vi "ReadDictionary.vi"(8 "error in (no error)":errorcluster, 11 "Dictionary File Path":path) -> (0 "error out":errorcluster, 1 "CSV String":string, 2 "Dictionary":T1, 3 "Dictionary File Path out":path)   [LabVIEW 2020]
uses:
  Dictionary--Cluster.ctl
  Font -- Cluster.ctl
  Phrase Dictionary Entry -- Cluster.ctl
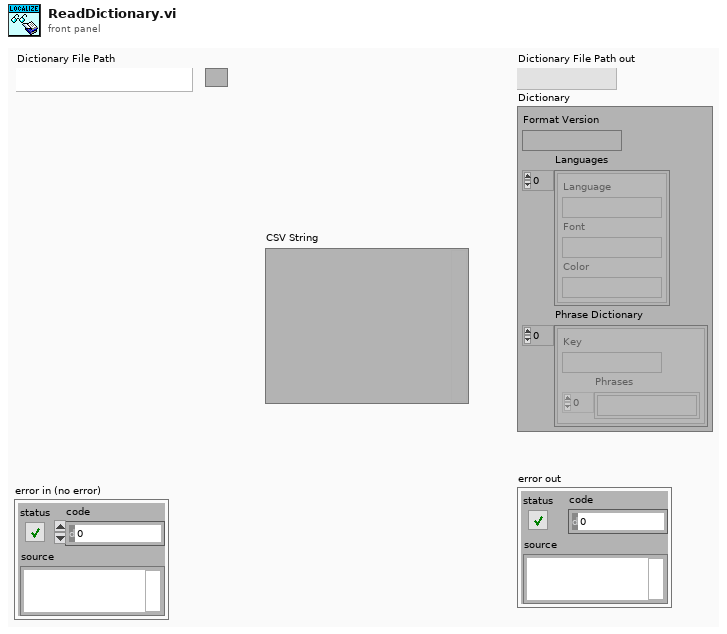
[diagram p1: front panel]
types:
  T1 = typedef "Dictionary--Cluster.ctl" = cluster{"Format Version":string, "Languages":T2[], "Phrase Dictionary":T3[]}
  T2 = typedef "Font -- Cluster.ctl" = cluster{"Language":string, "Font":string, "Color":string}
  T3 = typedef "Phrase Dictionary Entry -- Cluster.ctl" = cluster{"Key":string, "Phrases":string[]}
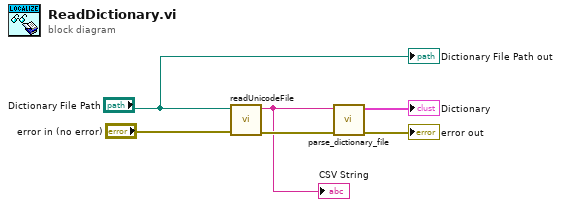
[diagram p0: block diagram]
diagram:
  n1 = call "readUnicodeFile.vi"("error in (no error)"="error in (no error)", "Unicode File Path"="Dictionary File Path") -> ("error out"=w4:errorcluster, "ASCII String"=w1:string)  [unwired: 8 in]
  "CSV String" <- w1
  n2 = call "parse_dictionary_file.vi"("error_in"=w4, "csv_string"=w1) -> ("error_out"=→"error out":errorcluster, "dictionary"=→"Dictionary":T1)  [unwired: 8 in]
  "Dictionary File Path out" <- "Dictionary File Path"
